vi "LibXML_SetAttribute.vi"(8 "error in":errorcluster, 9 "value":string, 10 "name":string, 11 "node":u32) -> (0 "error out":errorcluster, 3 "node copy out":u32)   [LabVIEW 2019, in "Tools.lvlib" / "LibXML.lvlib"]
doc: "Function: xmlSetProp\n\nxmlAttrPtr xmlSetProp (xmlNodePtr node, \n const xmlChar * name, \n const xmlChar * value)\n\nSet (or reset) an attribute carried by a node.\nnode: the node\nname: the attribute name\nvalue: the attribute value\nReturns: the attribute pointer."
uses:
  LibXML.lvlib
  dll/libxml2.dll
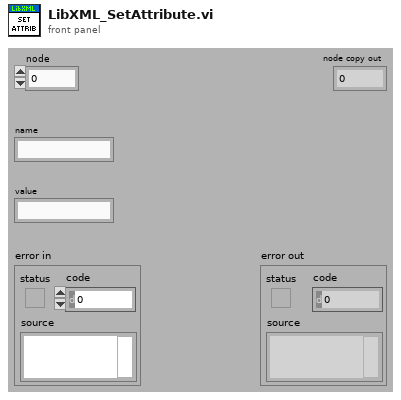
[diagram p1: front panel]
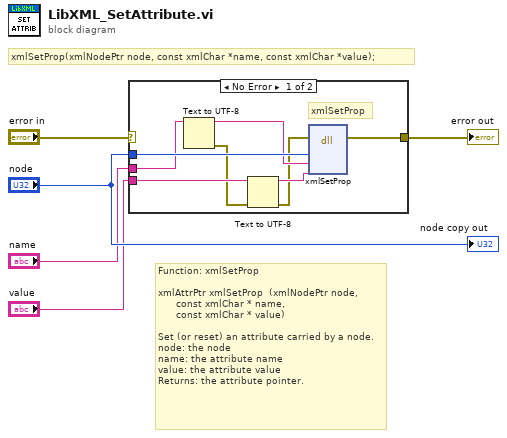
[diagram p0: block diagram]
diagram:
  # "Function: xmlSetProp\n\nxmlAttrPtr\txmlSetProp\t\t(xmlNodePtr node, \n\t\t\t\t\t const xmlChar * name, \n\t\t\t\t\t const xmlChar * value)\n\nSet (or reset) an attribute carried by a node.\nnode:\tthe node\nname:\tthe attribute name\nvalue:\tthe attribute value\nReturns:\tthe attribute pointer."
  # "xmlSetProp(xmlNodePtr node, const xmlChar *name, const xmlChar *value);"
  n1 = case shown="No Error" "error in" {
    selector: "error in" -> [_ w14]
    tunnel: [w12 w14] -> w4
    tunnel: "node" -> [w13 _]
    tunnel: "name" -> [w11 _]
    tunnel: "value" -> [w9 _]
    frame No Error {
      # "xmlSetProp"
      n2 = Text to UTF-8(11:w11) -> (0:w7:errorcluster, 3:w10:string)  [unwired: 2 in]
      n3 = Text to UTF-8(8:w7, 11:w9) -> (0:w6:errorcluster, 3:w8:string)  [unwired: 1 in]
      n4 = dll-call lib="C:/Projects/_Prywatne/MyCIT/Framework/Tools/XML/LibXML/dll/libxml2.dll" fn="xmlSetProp"(error in=w6, "node"=w13, "name"=w10, "value"=w8) -> (error out=w12:errorcluster)  [unwired: 6 in, 1 out]
    }
    frame Error {
    }
  }
  "error out" <- w4
  "node copy out" <- "node"
